vi "DAQ_Traffic_V2-1.vi"() -> ()   [LabVIEW 2021]
panel:
  out "YELLOW2":bool
  out "YELLOW1":bool
  out "GREEN2":bool
  out "GREEN1":bool
  out "RED2":bool
  out "RED1":bool
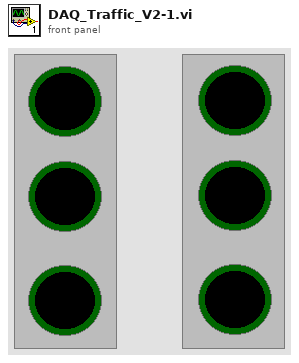
[diagram p1: front panel]
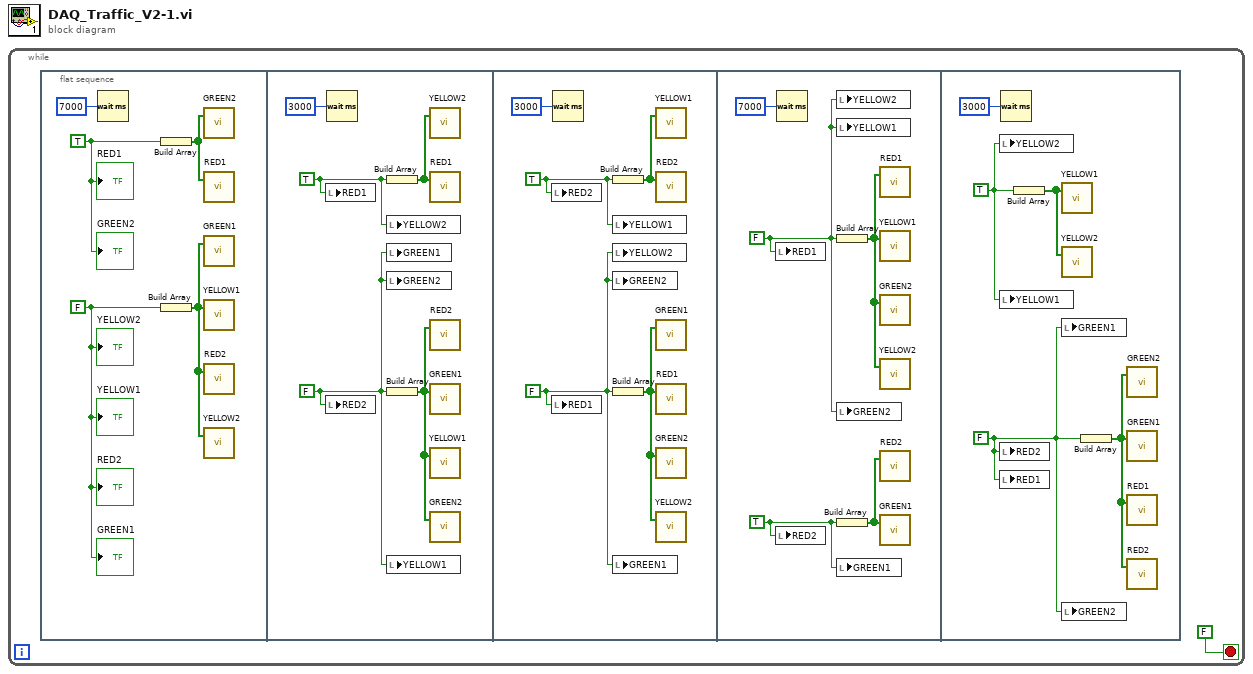
[diagram p0: block diagram]
diagram:
  n1 = while {
    stop <- FALSE stop-if-true
    n2 = flat-sequence {
      frame #0 {
        w3 = FALSE ("GREEN1")
        w5 = TRUE ("RED1")
        n3 = Wait (ms)(milliseconds to wait=u32 7000) -> ()  [unwired: 1 out]
        n4 = Build Array(w5) -> (w4:bool[])
        n5 = Build Array(w3) -> (w2:bool[])
        n6 = call "GREEN2"("data"=w4) -> ()  [unwired: 17 in, 2 out]
        n7 = call "RED1"("data"=w4) -> ()  [unwired: 17 in, 2 out]
        n8 = call "GREEN1"("data"=w2) -> ()  [unwired: 17 in, 2 out]
        n9 = call "YELLOW1"("data"=w2) -> ()  [unwired: 17 in, 2 out]
        n10 = call "RED2"("data"=w2) -> ()  [unwired: 17 in, 2 out]
        n11 = call "YELLOW2"("data"=w2) -> ()  [unwired: 17 in, 2 out]
        "RED1" <- w5
        "RED2" <- w3
        "GREEN1" <- w3
        "GREEN2" <- w5
        "YELLOW1" <- w3
        "YELLOW2" <- w3
      }
      frame #1 {
        w9 = FALSE ("YELLOW1")
        w10 = TRUE ("RED1")
        n12 = local write "RED1"(w10) -> ()
        n13 = local write "RED2"(w9) -> ()
        n14 = Wait (ms)(milliseconds to wait=u32 3000) -> ()  [unwired: 1 out]
        n15 = Build Array(w10) -> (w8:bool[])
        n16 = local write "YELLOW2"(w10) -> ()
        n17 = local write "GREEN1"(w9) -> ()
        n18 = local write "GREEN2"(w9) -> ()
        n19 = Build Array(w9) -> (w7:bool[])
        n20 = local write "YELLOW1"(w9) -> ()
        n21 = call "YELLOW2"("data"=w8) -> ()  [unwired: 17 in, 2 out]
        n22 = call "RED1"("data"=w8) -> ()  [unwired: 17 in, 2 out]
        n23 = call "RED2"("data"=w7) -> ()  [unwired: 17 in, 2 out]
        n24 = call "GREEN1"("data"=w7) -> ()  [unwired: 17 in, 2 out]
        n25 = call "YELLOW1"("data"=w7) -> ()  [unwired: 17 in, 2 out]
        n26 = call "GREEN2"("data"=w7) -> ()  [unwired: 17 in, 2 out]
      }
      frame #2 {
        w13 = FALSE ("RED1")
        w15 = TRUE ("RED2")
        n27 = local write "RED2"(w15) -> ()
        n28 = local write "RED1"(w13) -> ()
        n29 = Wait (ms)(milliseconds to wait=u32 3000) -> ()  [unwired: 1 out]
        n30 = Build Array(w15) -> (w14:bool[])
        n31 = local write "YELLOW1"(w15) -> ()
        n32 = local write "YELLOW2"(w13) -> ()
        n33 = local write "GREEN2"(w13) -> ()
        n34 = Build Array(w13) -> (w12:bool[])
        n35 = local write "GREEN1"(w13) -> ()
        n36 = call "YELLOW1"("data"=w14) -> ()  [unwired: 17 in, 2 out]
        n37 = call "RED2"("data"=w14) -> ()  [unwired: 17 in, 2 out]
        n38 = call "GREEN1"("data"=w12) -> ()  [unwired: 17 in, 2 out]
        n39 = call "RED1"("data"=w12) -> ()  [unwired: 17 in, 2 out]
        n40 = call "GREEN2"("data"=w12) -> ()  [unwired: 17 in, 2 out]
        n41 = call "YELLOW2"("data"=w12) -> ()  [unwired: 17 in, 2 out]
      }
      frame #3 {
        w18 = FALSE ("YELLOW1")
        w20 = TRUE ("RED2")
        n42 = local write "RED1"(w18) -> ()
        n43 = local write "RED2"(w20) -> ()
        n44 = Wait (ms)(milliseconds to wait=u32 7000) -> ()  [unwired: 1 out]
        n45 = local write "YELLOW2"(w18) -> ()
        n46 = local write "YELLOW1"(w18) -> ()
        n47 = Build Array(w18) -> (w17:bool[])
        n48 = local write "GREEN2"(w18) -> ()
        n49 = Build Array(w20) -> (w19:bool[])
        n50 = local write "GREEN1"(w20) -> ()
        n51 = call "RED1"("data"=w17) -> ()  [unwired: 17 in, 2 out]
        n52 = call "YELLOW1"("data"=w17) -> ()  [unwired: 17 in, 2 out]
        n53 = call "GREEN2"("data"=w17) -> ()  [unwired: 17 in, 2 out]
        n54 = call "YELLOW2"("data"=w17) -> ()  [unwired: 17 in, 2 out]
        n55 = call "RED2"("data"=w19) -> ()  [unwired: 17 in, 2 out]
        n56 = call "GREEN1"("data"=w19) -> ()  [unwired: 17 in, 2 out]
      }
      frame #4 {
        w23 = FALSE ("GREEN2")
        w25 = TRUE ("YELLOW2")
        n57 = local write "YELLOW2"(w25) -> ()
        n58 = local write "YELLOW1"(w25) -> ()
        n59 = local write "RED2"(w23) -> ()
        n60 = local write "RED1"(w23) -> ()
        n61 = Wait (ms)(milliseconds to wait=u32 3000) -> ()  [unwired: 1 out]
        n62 = Build Array(w25) -> (w24:bool[])
        n63 = call "YELLOW1"("data"=w24) -> ()  [unwired: 17 in, 2 out]
        n64 = call "YELLOW2"("data"=w24) -> ()  [unwired: 17 in, 2 out]
        n65 = local write "GREEN1"(w23) -> ()
        n66 = local write "GREEN2"(w23) -> ()
        n67 = Build Array(w23) -> (w22:bool[])
        n68 = call "GREEN2"("data"=w22) -> ()  [unwired: 17 in, 2 out]
        n69 = call "GREEN1"("data"=w22) -> ()  [unwired: 17 in, 2 out]
        n70 = call "RED1"("data"=w22) -> ()  [unwired: 17 in, 2 out]
        n71 = call "RED2"("data"=w22) -> ()  [unwired: 17 in, 2 out]
      }
    }
  }
